vi "Publish to Topic.vi"(8 "error in":errorcluster, 10 "Topic.lvclass":refnum<class "Topic.lvclass">, 11 "Client in":refnum<class "Client.lvclass">) -> (0 "error out":errorcluster, 3 "Client out":refnum<class "Client.lvclass">)   [LabVIEW 2014, in "Client.lvclass"]
uses:
  Client.lvclass
  Topic_class/Topic.lvclass
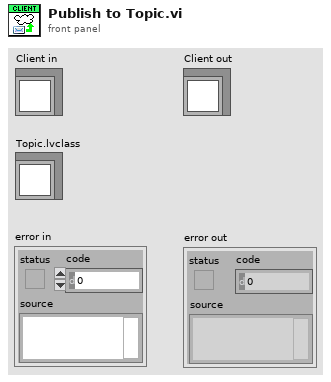
[diagram p1: front panel]
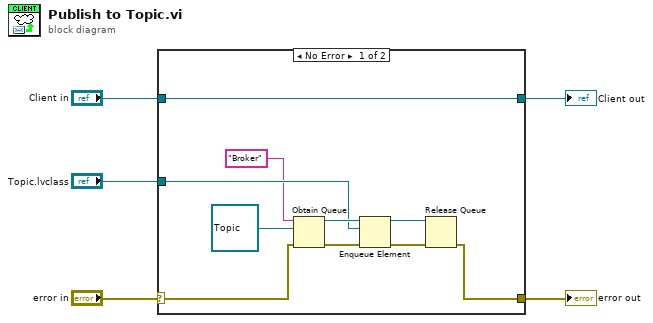
[diagram p0: block diagram]
diagram:
  n1 = case shown="No Error" "error in" {
    selector: "error in" -> [w8 w17]
    tunnel: [w7 w17] -> w4
    tunnel: [w15 w16] -> w2
    tunnel: "Client in" -> [w15 w16]
    tunnel: "Topic.lvclass" -> [w9 _]
    frame No Error {
      n2 = Obtain Queue(name (unnamed)="Broker" ("Client ID"), element data type=refnum<class "Topic.lvclass"> refnum ("Topic.lvclass"), error in (no error)=w8) -> (queue out=w11:refnum<queue>, error out=w13:errorcluster)  [unwired: 2 in, 1 out]
      n3 = Enqueue Element(queue=w11, element=w9, error in (no error)=w13) -> (queue out=w12:refnum<queue>, error out=w14:errorcluster)  [unwired: 1 in, 1 out]
      n4 = Release Queue(queue=w12, error in (no error)=w14) -> (error out=w7:errorcluster)  [unwired: 1 in, 2 out]
    }
    frame Error {
    }
  }
  "error out" <- w4
  "Client out" <- w2
